vi "GA_FitnessOnTestData.vi"(0 "ClassifierClass.lvclass":refnum<class "ClassifierClass.lvclass">, 1 "Phenotype":i8[](array[numeric]), 2 "TrainingData":T1, 3 "TestData":T1=enum."Test Data") -> (5 "Fitness":dbl)   [LabVIEW 2016, in "GA.lvlib"]
uses:
  GA.lvlib
  4. Accuracy Assessment for EEG Classification/_vlib/ClassifierClass.lvclass
  4. Accuracy Assessment for EEG Classification/_vlib/CU_DataTypes.ctl
  4. Accuracy Assessment for EEG Classification/Classifier.lvlib
panel:
  # "This VI is a part of BCI Design library, http://www.ru-bci.org \nCopyright © 2020, Sotnikov Peter, All rights reserved. License: GNU GPLv3"
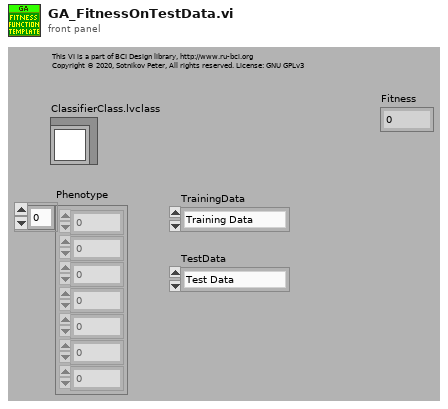
[diagram p1: front panel]
types:
  T1 = typedef "Classifier.lvlib/CU_DataTypes.ctl" = enum16{"Training Data", "Test Data", "Training Data (cross-check)", "Test Data (cross-check)"}
  T2 = typedef "Classifier.lvlib/CU_ClassifierTypes.ctl" = enum16{"Multilayer perceptron", "k NN Classifier", "SVM Committee", "Mahalanobis distance", "SVM Classifier"}
  T3 = typedef "IMAQ Classifier Session.ctl" = refnum<k1>
  T4 = typedef "NILabs_MLT.lvlib/ml_BP_Project.ctl" = cluster{"Training Data":T5, "Normalize Info":T6, "3-layer NN":T7, "Ternimal Condition":T8}
  T5 = typedef "NILabs_MLT.lvlib/ml_BP_Data.ctl" = cluster{"dim in":i32, "dim out":i32, "# samples":i32, "Input":dbl[][], "Output":dbl[][]}
  T6 = typedef "NILabs_MLT.lvlib/ml_BP_Normalize Data.ctl" = cluster{"input min":dbl[], "input max":dbl[], "output min":dbl[], "output max":dbl[]}
  T7 = typedef "NILabs_MLT.lvlib/ml_BP_3layer Feedforward.ctl" = cluster{"# input neuron ":i32, "# hidden neuron":i32, "# output neuron":i32, "Weight (I->H)":dbl[][], "Weight (H->O)":dbl[][], "Output":dbl[][], "Hidden Out":dbl[][], "Derivation Output":dbl[][], "Derivation Hidden":dbl[][], "dw (I->H)":dbl[][], "dw (H->O)":dbl[][]}
  T8 = typedef "NILabs_MLT.lvlib/ml_BP_Terminal Condition.ctl" = cluster{"min MSE":dbl, "min delta MSE":dbl, "min step length":dbl, "max iteration":dbl}
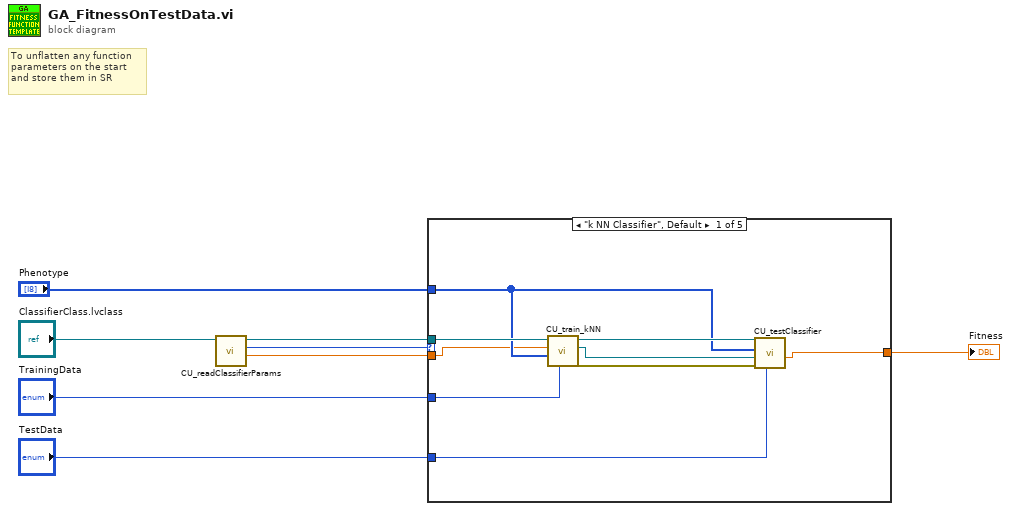
[diagram p0: block diagram]
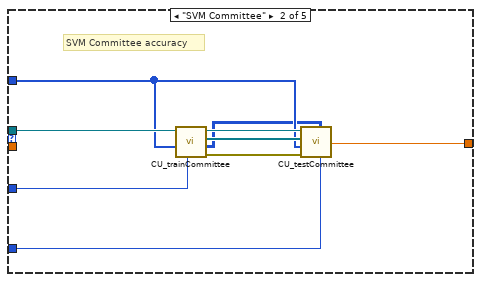
[diagram p2: hidden frame]
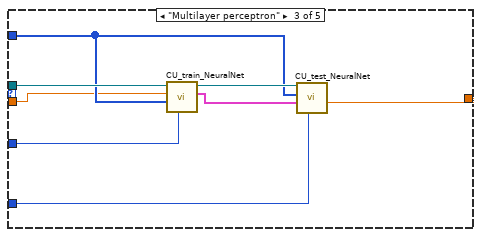
[diagram p3: hidden frame]
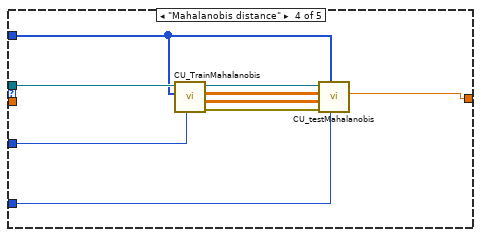
[diagram p4: hidden frame]
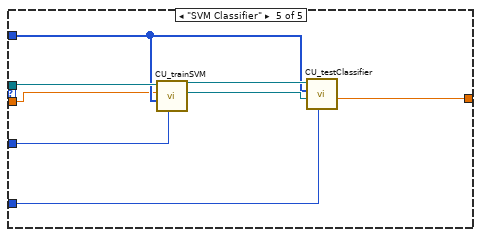
[diagram p5: hidden frame]
diagram:
  # "To unflatten any function\nparameters on the start\nand store them in SR"
  n1 = call-dynamic "CU_readClassifierParams.vi"("ClassifierClass in"="ClassifierClass.lvclass") -> ("Classifier Metaparameter out"=w1:dbl, "ClassifierType out"=w7:T2, "ClassifierClass out"=w8:refnum<class "ClassifierClass.lvclass">)  [unwired: 7 in, 1 out]
  n2 = case shown="\"k NN Classifier\", Default" w7 {
    tunnel: w8 -> [w17 w26 w34 w43 w51]
    tunnel: [w12 w21 w30 w35 w45] -> w2
    tunnel: "Phenotype" -> [w14 w22 w31 w36 w46]
    tunnel: "TrainingData" -> [w11 w19 w29 w41 w50]
    tunnel: "TestData" -> [w10 w18 w28 w40 w49]
    tunnel: w1 -> [w9 _ w27 _ w44]
    frame "k NN Classifier", Default {
      n3 = call "CU_train_kNN.vi"("DataTypes"=w11, "Indices"=w14, "k value"=w9, "ClassifierClass in"=w17) -> ("error out"=w13:errorcluster, "Classifier Session out"=w15:T3, "ClassifierClass out"=w16:refnum<class "ClassifierClass.lvclass">)  [unwired: 5 in]
      n4 = call "CU_testClassifier.vi"("DataTypes"=w10, "error in"=w13, "Classifier Session Ref"=w15, "Indices"=w14, "ClassifierClass in"=w16) -> ("Accuracy"=w12:dbl)  [unwired: 3 in, 3 out]
    }
    frame "SVM Committee" {
      # "SVM Committee accuracy"
      n5 = call "CU_trainCommittee.vi"("DataTypes"=w19, "Indices"=w22, "ClassifierClass in"=w26) -> ("error out"=w24:errorcluster, "Classification Distribution"=w20:i32[][][], "Classifier Refs out"=w23:T3[], "ClassifierClass out"=w25:refnum<class "ClassifierClass.lvclass">)  [unwired: 5 in]
      n6 = call "CU_testCommittee.vi"("ClassifierClass in"=w25, "Classifier Refs in"=w23, "Indices"=w22, "error in"=w24, "Classification Distribution"=w20, "DataTypes"=w18) -> ("Accuracy"=w21:dbl)  [unwired: 3 out]
    }
    frame "Multilayer perceptron" {
      n7 = call "CU_train_NeuralNet.vi"("DataTypes"=w29, "Indices"=w31, "# of hidden neuron"=w27, "ClassifierClass in"=w34) -> ("ANN out"=w32:T4, "ClassifierClass out"=w33:refnum<class "ClassifierClass.lvclass">)  [unwired: 4 in, 2 out]
      n8 = call "CU_test_NeuralNet.vi"("DataTypes"=w28, "ANN in"=w32, "Indices"=w31, "ClassifierClass in"=w33) -> ("Accuracy"=w30:dbl)  [unwired: 4 in, 3 out]
    }
    frame "Mahalanobis distance" {
      n9 = call "CU_TrainMahalanobis.vi"("DataTypes"=w41, "Indices"=w36, "ClassifierClass in"=w43) -> ("error out"=w39:errorcluster, "Mean vectors"=w38:dbl[][], "Covariance matricies"=w37:dbl[][][], "ClassifierClass out"=w42:refnum<class "ClassifierClass.lvclass">)  [unwired: 5 in]
      n10 = call "CU_testMahalanobis.vi"("DataTypes"=w40, "Indices"=w36, "error in"=w39, "Mean vectors"=w38, "Covariance matricies"=w37, "ClassifierClass in"=w42) -> ("Accuracy"=w35:dbl)  [unwired: 2 in, 3 out]
    }
    frame "SVM Classifier" {
      n11 = call "CU_trainSVM.vi"("Train Data"=w50, "Indices"=w46, "Nu Value"=w44, "ClassifierClass in"=w51) -> ("Classifier Session out"=w47:T3, "ClassifierClass out"=w48:refnum<class "ClassifierClass.lvclass">)  [unwired: 5 in, 1 out]
      n12 = call "CU_testClassifier.vi"("DataTypes"=w49, "Classifier Session Ref"=w47, "Indices"=w46, "ClassifierClass in"=w48) -> ("Accuracy"=w45:dbl)  [unwired: 4 in, 3 out]
    }
  }
  "Fitness" <- w2
